vi "test7-AsyncMessageWithoutReply.vi"(8 "error in (no error)":errorcluster, 11 "TestCase in":refnum<class "testcase-CSMMessage.lvclass">) -> (0 "error out":errorcluster, 3 "TestCase out":refnum<class "testcase-CSMMessage.lvclass">)   [LabVIEW 2017, in "testcase-CSMMessage.lvclass"]
uses:
  testcase-CSMMessage.lvclass
  7412589e-de49-4983-aece-358686b48526.vi
  <vilib>/addons/_JKI Toolkits/VI Tester/TestCase.llb/TestCase.lvclass
  src/user.lib/_NEVSTOP/Communicable State Machine(CSM)/Communicable State Machine.lvlib
  C:/Program Files (x86)/National Instruments/LabVIEW 2017/vi.lib/addons/_JKI Toolkits/VI Tester/TestCase.llb/TestCase.lvclass
panel:
  out "Loop count":i32
  out "concatenated string":string
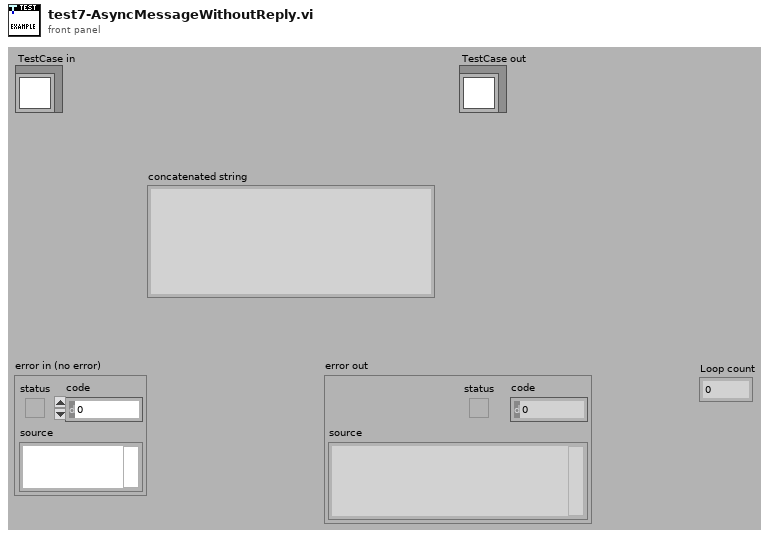
[diagram p1: front panel]
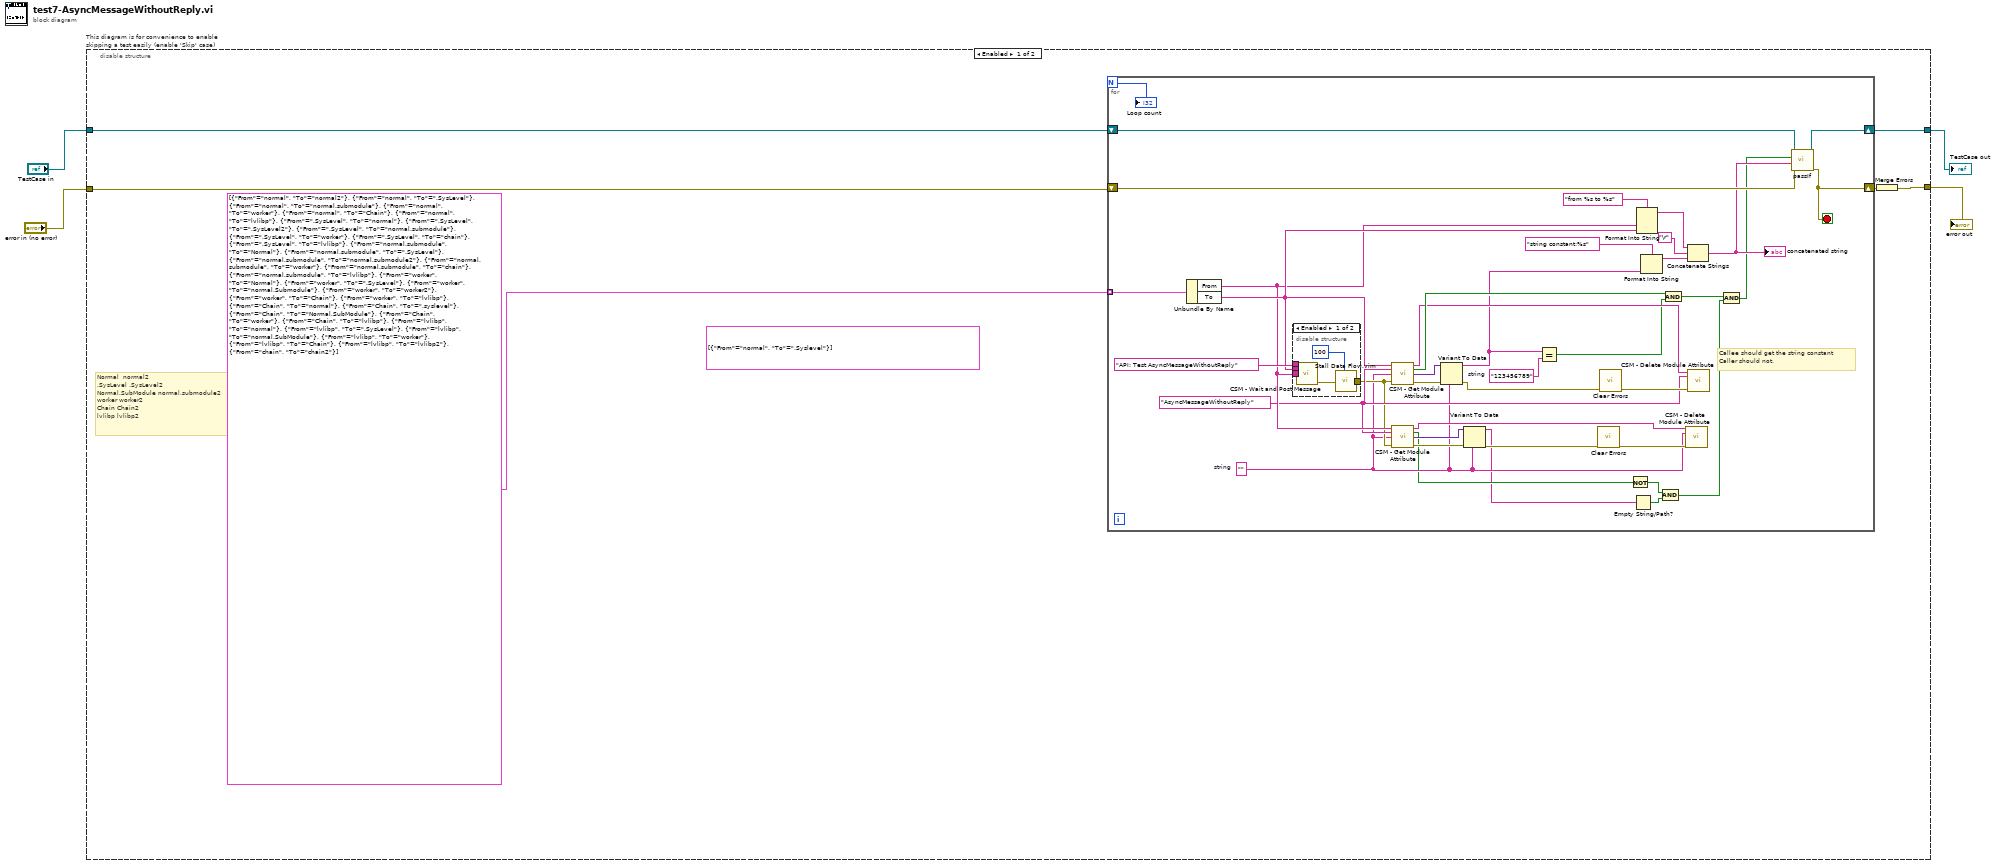
[diagram p0: block diagram]
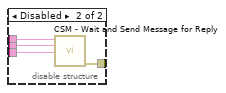
[diagram p2: hidden frame]
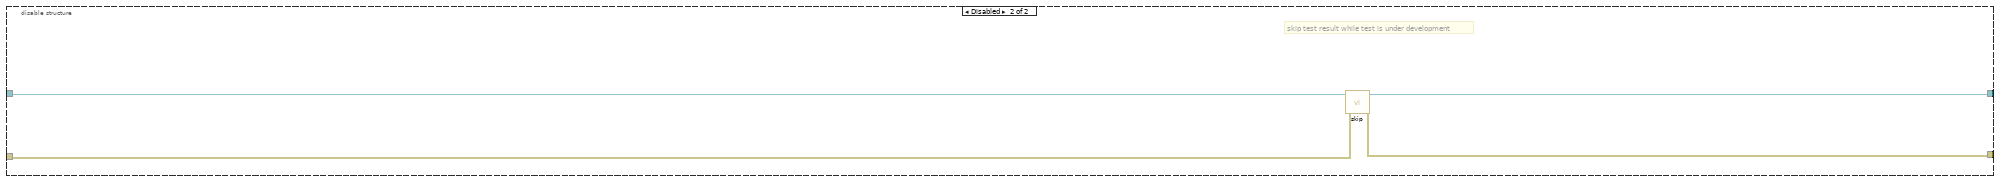
[diagram p3: hidden frame]
diagram:
  n1 = disable-structure "This diagram is for convenience to enable skipping a test easily (enable 'Skip' case)" shown="Enabled" {
    disable-tunnel: "TestCase in" -> [w10 w63]
    disable-tunnel: [w9 w61] -> w1
    disable-tunnel: [w6 w62] -> w3
    disable-tunnel: "error in (no error)" -> [w7 w60]
    frame Enabled {
      (unwired) cluster{"From":string, "To":string}[] [{"From"="normal", "To"=".Syslevel"}]
      # "Normal  normal2\n.SysLevel .SysLevel2\nNormal.SubModule normal.submodule2\nworker worker2\nChain Chain2\nlvlibp lvlibp2"
      n2 = for {
        N -> [w31]
        tunnel: cluster{"From":string, "To":string}[] [{"From"="normal", "To"="normal2"}, {"From"="normal", "To"=".SysLevel"}, {"From"="normal", "To"="normal.submodule"}, {"From"="normal", "To"="worker"}, {"From"="normal", "To"="Chain"}, {"From"="normal", "To"="lvlibp"}, {"From"=".SysLevel", "To"="normal"}, {"From"=".SysLevel", "To"=".SysLevel2"}, {"From"=".SysLevel", "To"="normal.submodule"}, {"From"=".SysLevel", "To"="worker"}, {"From"=".SysLevel", "To"="chain"}, {"From"=".SysLevel", "To"="lvlibp"}, {"From"="normal.submodule", "To"="Normal"}, {"From"="normal.submodule", "To"=".SysLevel"}, {"From"="normal.submodule", "To"="normal.submodule2"}, {"From"="normal.submodule", "To"="worker"}, {"From"="normal.submodule", "To"="chain"}, {"From"="normal.submodule", "To"="lvlibp"}, {"From"="worker", "To"="Normal"}, {"From"="worker", "To"=".SysLevel"}, {"From"="worker", "To"="normal.Submodule"}, {"From"="worker", "To"="worker2"}, {"From"="worker", "To"="Chain"}, {"From"="worker", "To"="lvlibp"}, {"From"="Chain", "To"="normal"}, {"From"="Chain", "To"=".syslevel"}, {"From"="Chain", "To"="Normal.SubModule"}, {"From"="Chain", "To"="worker"}, {"From"="Chain", "To"="lvlibp"}, {"From"="lvlibp", "To"="normal"}, {"From"="lvlibp", "To"=".SysLevel"}, {"From"="lvlibp", "To"="normal.SubModule"}, {"From"="lvlibp", "To"="worker"}, {"From"="lvlibp", "To"="Chain"}, {"From"="lvlibp", "To"="lvlibp2"}, {"From"="chain", "To"="chain2"}] -> [w42] mode=indexing
        shift-right: [w48] -> w9
        shift-left: w10 -> [w49]
        shift-right: [w32] -> w8
        shift-left: w7 -> [w47]
        stop <- w32 stop-if-true
        w28 = "123456789"  # string
        w18 = ""  # string
        w25 = "AsyncMessageWithoutReply" ("State With Arguments")
        # "Callee should get the string constant\nCaller should not."
        n3 = Unbundle By Name(w42) -> ("From"=w26:string, "To"=w30:string)
        n4 = disable-structure shown="Enabled" {
          disable-tunnel: "API: Test AsyncMessageWithoutReply" ("State") -> [w55 w58]
          disable-tunnel: w30 -> [w54 w57]
          disable-tunnel: w26 -> [w53 w56]
          disable-tunnel: [w51 w59] -> w24
          frame Enabled {
            n5 = call "CSM - Wait and Post Message.vi"("State"=w55, "Arguments (\"\")"=w54, "Target Module"=w53) -> ("error out"=w52:errorcluster)  [unwired: 12 in]
            n6 = call "Stall Data Flow.vim"("value in"=w52, "milliseconds to wait"=u32 100) -> ("value out"=w51:errorcluster)  [unwired: 1 out]
          }
          frame Disabled {
            n7 = call "CSM - Wait and Send Message for Reply.vi"("State"=w58, "Arguments (\"\")"=w57, "Target Module"=w56) -> ("error out"=w59:errorcluster)  [unwired: 10 in, 2 out]
          }
        }
        n8 = call "CSM - Get Module Attribute.vi"("CSM Name"=w30, "Attribute"=w25, "Default Value (Empty Variant)"=w18, "Error In"=w24) -> ("CSM Name (Dup)"=w40:string, "Found"=w43:bool, "Value"=w44:variant, "error out"=w45:errorcluster)  [unwired: 7 in, 1 out]
        n9 = call "CSM - Get Module Attribute.vi"("CSM Name"=w26, "Attribute"=w25, "Default Value (Empty Variant)"=w18, "Error In"=w24) -> ("CSM Name (Dup)"=w19:string, "Found"=w17:bool, "Value"=w20:variant, "error out"=w23:errorcluster)  [unwired: 7 in, 1 out]
        n10 = Variant To Data(error in=w45, type=w18, Variant=w44) -> (data=w27:string, error out=w34:errorcluster)
        n11 = Variant To Data(error in=w23, type=w18, Variant=w20) -> (data=w16:string, error out=w22:errorcluster)
        n12 = Equal?(x=w27, y=w28) -> (x = y?=w29:bool)
        n13 = call <vilib>:"Clear Errors.vi"("error in (no error)"=w22) -> ("error out"=w21:errorcluster)  [unwired: 5 in, 1 out]
        n14 = call <vilib>:"Clear Errors.vi"("error in (no error)"=w34) -> ("error out"=w33:errorcluster)  [unwired: 5 in, 1 out]
        n15 = Not(x=w17) -> (.not. x?=w13:bool)
        n16 = Empty String/Path?(string/path=w16) -> (empty?=w15:bool)
        n17 = Format Into String(format string="from %s to %s", w26, w30) -> (resulting string=w36:string)  [unwired: 2 in, 1 out]
        n18 = Format Into String(format string="string constant:%s", w27) -> (resulting string=w39:string)  [unwired: 2 in, 1 out]
        n19 = And(x=w13, y=w15) -> (x .and. y?=w11:bool)
        n20 = And(x=w43, y=w29) -> (x .and. y?=w14:bool)
        n21 = call "CSM - Delete Module Attribute.vi"("CSM Name"=w19, "Attribute"=w18, "Error In"=w21) -> ()  [unwired: 9 in, 4 out]
        n22 = Concatenate Strings(w36, "\r", w39) -> (w37:string)
        "concatenated string" <- w37
        n23 = call "CSM - Delete Module Attribute.vi"("CSM Name"=w40, "Attribute"=w25, "Error In"=w33) -> ()  [unwired: 9 in, 4 out]
        n24 = And(x=w14, y=w11) -> (x .and. y?=w12:bool)
        n25 = call-dynamic "passIf.vi"("error in (no error)"=w47, "message (\"\")"=w37, "pass"=w12, "TestCase in"=w49) -> ("error out"=w32:errorcluster, "TestCase out"=w48:refnum<class "testcase-CSMMessage.lvclass">)  [unwired: 6 in]
        "Loop count" <- w31
      }
      n26 = Merge Errors(w8) -> (w6:errorcluster)
    }
    frame Disabled {
      # "skip test result while test is under development"
      n27 = call <vilib>:"skip.vi"("error in (no error)"=w60, "TestCase in"=w63) -> ("error out"=w62:errorcluster, "TestCase out"=w61:refnum<class "testcase-CSMMessage.lvclass">)  [unwired: 8 in]
    }
  }
  "error out" <- w3
  "TestCase out" <- w1
